vi "Coerce selector control value.vi"(6 "New strings[]":string[](array[string]), 7 "String of currently selected item":string, 9 "#of selected ROI":i32, 11 "Set selection to index 0":bool) -> (2 "Selection index out":u16)   [LabVIEW 2020]
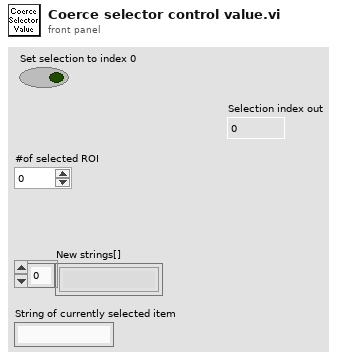
[diagram p1: front panel]
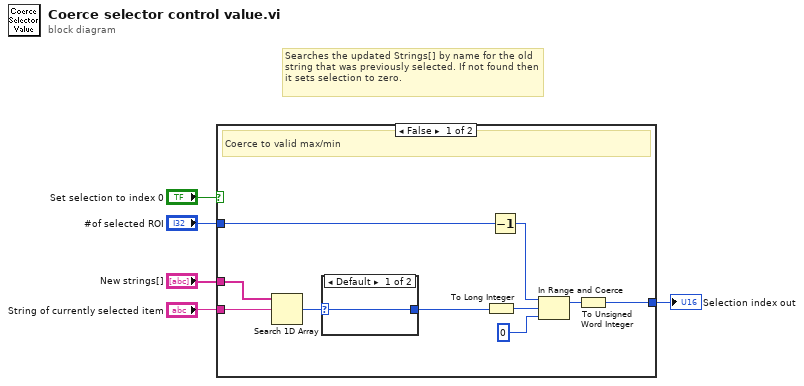
[diagram p0: block diagram]
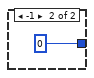
[diagram p2: hidden frame]
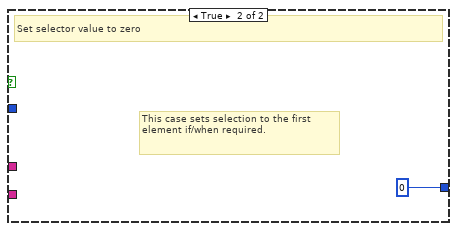
[diagram p3: hidden frame]
diagram:
  # "Searches the updated Strings[] by name for the old string that was previously selected. If not found then it sets selection to zero."
  n1 = case shown="False" "Set selection to index 0" {
    tunnel: "#of selected ROI" -> [w6 _]
    tunnel: [w11 u16 0 ("lower limit")] -> w4
    tunnel: "New strings[]" -> [w9 _]
    tunnel: "String of currently selected item" -> [w8 _]
    frame False {
      # "Coerce to valid max/min"
      n2 = Search 1D Array(1D array=w9, element=w8) -> (index of element=w10:i32)  [unwired: 1 in]
      n3 = case shown="Default" w10 {
        selector: w10 -> [w16 _]
        tunnel: [w16 0] -> w7
        frame Default {
        }
        frame -1 {
        }
      }
      n4 = To Long Integer(number=w7) -> (32bit integer=w12:i32)
      n5 = Decrement(x=w6) -> (x-1=w15:i32)
      n6 = In Range and Coerce(upper limit=w15, x=w12, lower limit=0) -> (coerced(x)=w14:i32)  [unwired: 1 out]
      n7 = To Unsigned Word Integer(number=w14) -> (unsigned 16bit integer=w11:u16)
    }
    frame True {
      # "This case sets selection to the first element if/when required."
      # "Set selector value to zero"
    }
  }
  "Selection index out" <- w4
